vi "Set deceleration DSP402.vi"(8 "error in (no error)":errorcluster, 10 "Deceleration units":u32, 11 "DSP402 in":refnum<class "DSP402.lvclass">) -> (0 "error out":errorcluster, 3 "DSP402 out":refnum<class "DSP402.lvclass">)   [LabVIEW 2017, in "canopen.lvlib" / "DSP402.lvclass"]
uses:
  DSP402.lvclass
  DSP402.lvclass/DSP402.ctl
  CANopen/Multiplexor.ctl
  Download DSP402 (U32).vi
  CANopen/CANopen.lvclass
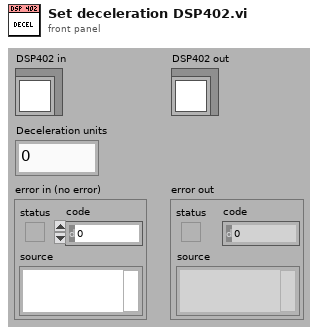
[diagram p1: front panel]
types:
  T1 = typedef "canopen.lvlib/DSP402.lvclass/DriveMode.ctl" = i8
  T2 = typedef "canopen.lvlib/CANopen.lvclass/Multiplexor.ctl" = cluster{"Index":u16, "Sub-index":u8}
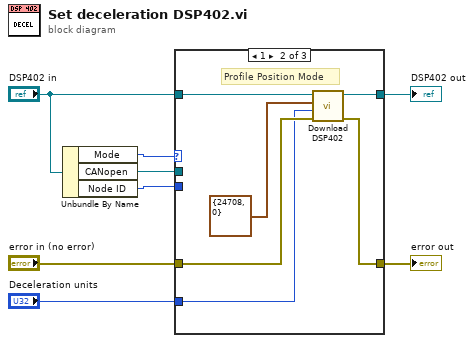
[diagram p0: block diagram]
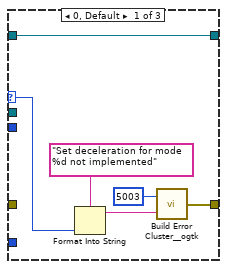
[diagram p2: hidden frame]
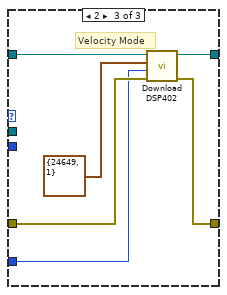
[diagram p3: hidden frame]
diagram:
  n1 = Unbundle By Name("DSP402 in") -> ("Mode"=w3:T1, "CANopen"=w6:refnum<class "CANopen.lvclass">, "Node ID"=w5:u8)
  n2 = case shown="1" w3 {
    selector: w3 -> [w11 _ _]
    tunnel: [w12 w19 w25] -> w4
    tunnel: "error in (no error)" -> [_ w18 w24]
    tunnel: "Deceleration units" -> [_ w17 w23]
    tunnel: w6 -> [_ _ _]
    tunnel: w5 -> [_ _ _]
    tunnel: [w9 w15 w21] -> w2
    tunnel: "DSP402 in" -> [w9 w16 w22]
    frame 0, Default {
      n3 = Format Into String(format string="Set deceleration for mode %d not implemented", w11) -> (resulting string=w13:string)  [unwired: 2 in, 1 out]
      n4 = call <userlib>:"Build Error Cluster__ogtk.vi"("String to Prepend to source (\"\")"=w13, "code"=5003) -> ("error out"=w12:errorcluster)
    }
    frame 1 {
      # "Profile Position Mode"
      n5 = call-poly "Download DSP402.vi"("error in (no error)"=w18, "Value"=w17, "Multiplexor"=T2 {"Index"=24708, "Sub-index"=0}, "DSP402 in"=w16) -> ("error out"=w19:errorcluster, "DSP402 out"=w15:refnum<class "DSP402.lvclass">)  [unwired: 1 in, 1 out]
    }
    frame 2 {
      # "Velocity Mode"
      n6 = call-poly "Download DSP402.vi"("error in (no error)"=w24, "Value"=w23, "Multiplexor"=T2 {"Index"=24649, "Sub-index"=1}, "DSP402 in"=w22) -> ("error out"=w25:errorcluster, "DSP402 out"=w21:refnum<class "DSP402.lvclass">)  [unwired: 2 out]
    }
  }
  "error out" <- w4
  "DSP402 out" <- w2
